vi "AddGlyphtoGManager.vi"(8 "error in":errorcluster, 10 "glyph manager":T1, 11 "CEF_serializable node in":refnum<class "CEF_serializable node.lvclass">) -> (0 "error out":errorcluster, 2 "glyph manager out":T1, 3 "CEF_serializable node out":refnum<class "CEF_serializable node.lvclass">)   [LabVIEW 2023, in "CEF.lvlib" / "CEF_serializable node.lvclass"]
doc: "Copyright 2017 National Instruments Corporation\n\nLicensed under the Apache License, Version 2.0 (the \"License\"); you may not use this file except in compliance with the License. You may obtain a copy of the License at http://www.apache.org/licenses/LICENSE-2.0\nUnless required by applicable law or agreed to in writing, software distributed under the License is distributed on an \"AS IS\" BASIS, WITHOUT WARRANTIES OR CONDITIONS OF ANY KIND, either express or implied. See the License for the specific language governing permissions and limitations under the License."
uses:
  CEF_serializable node.lvclass
  glyph manager/glyph manager.ctl
  <vilib>/picture/picture.llb/imagedata.ctl
  Node/CEF_Node.lvclass
  CEF.lvlib
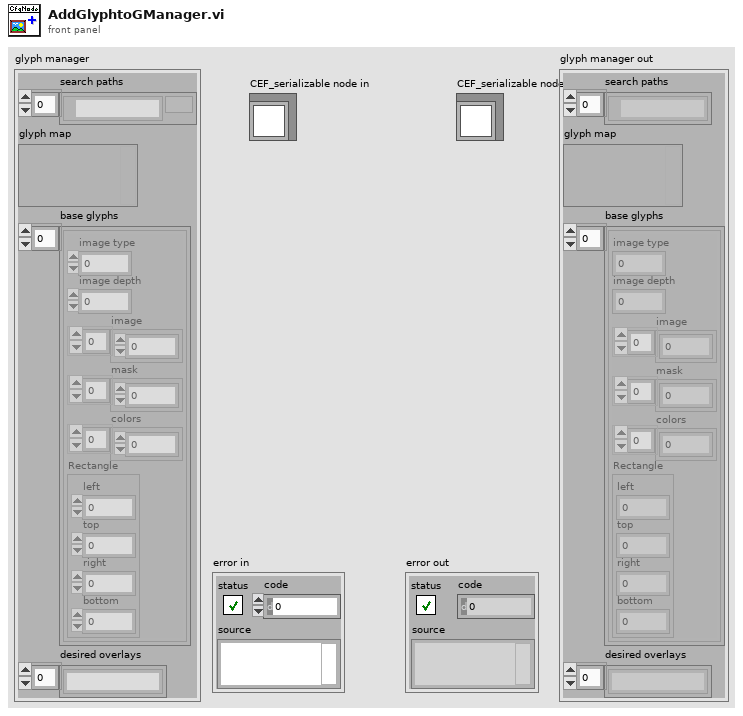
[diagram p1: front panel]
types:
  T1 = typedef "CEF.lvlib/glyph manager.ctl" = cluster{"search paths":path[], "glyph map":variant, "base glyphs":T2[], "desired overlays":string[]}
  T2 = typedef "imagedata.ctl" = cluster{"image type":i32, "image depth":i32, "image":u8[], "mask":u8[], "colors":u32[], "Rectangle":cluster{"left":i16, "top":i16, "right":i16, "bottom":i16}}
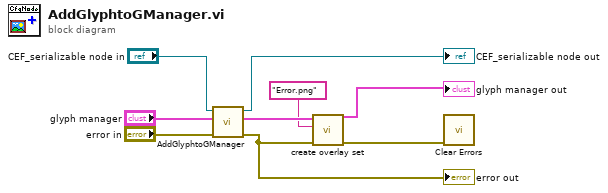
[diagram p0: block diagram]
diagram:
  n1 = call-parent "AddGlyphtoGManager.vi"("error in"="error in", "glyph manager"="glyph manager", "CEF_Node in"="CEF_serializable node in") -> ("error out"=w3:errorcluster, "glyph manager out"=w5:T1, "CEF_Node out"=→"CEF_serializable node out":refnum<class "CEF_serializable node.lvclass">)  [unwired: 6 in]
  "error out" <- w3
  n2 = call "create overlay set.vi"("error in"=w3, "overlay glyph"="Error.png", "glyph manager in"=w5) -> ("error out"=w2:errorcluster, "glyph manager out"=→"glyph manager out":T1)  [unwired: 7 in]
  n3 = call <vilib>:"Clear Errors.vi"("error in (no error)"=w2) -> ()  [unwired: 5 in, 2 out]
